vi "iteration_counter.vi"(1 "ms per iteration":i32, 2 "index":i32) -> (0 "seconds":i32)   [LabVIEW 2010]
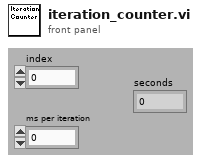
[diagram p1: front panel]
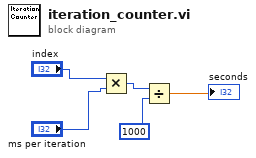
[diagram p0: block diagram]
diagram:
  n1 = Multiply(x="index", y="ms per iteration") -> (x*y=w3:i32)
  n2 = Divide(x=w3, y=1000) -> (x/y=→"seconds":dbl)
